vi "Read Results from processing.vi"(8 "error in":errorcluster, 11 "Conversion runtime in":refnum<class "Conversion runtime.lvclass">) -> (0 "error out":errorcluster, 2 "Results from processing":T1, 3 "Conversion runtime out":refnum<class "Conversion runtime.lvclass">)   [LabVIEW 2017, in "Conversion runtime.lvclass"]
uses:
  Conversion runtime.lvclass
  configuration/result data indices.ctl
  Conversion runtime.lvclass/Conversion runtime.ctl
  configuration/Conversion configuration.lvclass
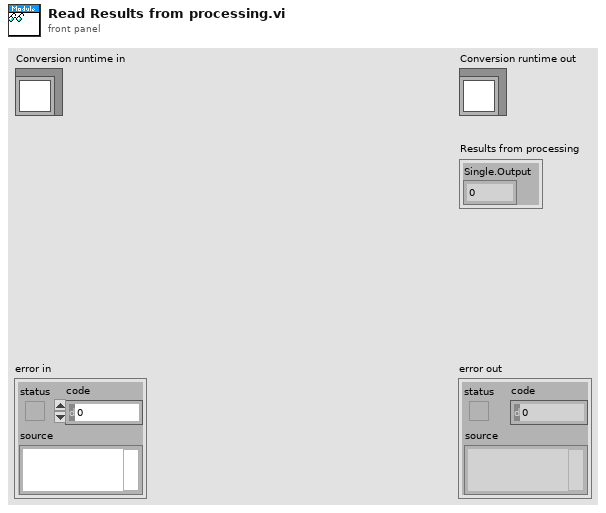
[diagram p1: front panel]
types:
  T1 = typedef "Conversion configuration.lvclass/result data indices.ctl" = cluster{"Single.Output":i32}
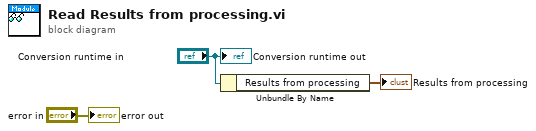
[diagram p0: block diagram]
diagram:
  n1 = Unbundle By Name("Conversion runtime in") -> ("Results from processing"=→"Results from processing":T1)
  "error out" <- "error in"
  "Conversion runtime out" <- "Conversion runtime in"
